vi "Write.vi"(8 "error in (no error)":errorcluster, 11 "UI VISA Terminal in":refnum<class "UI VISA Terminal.lvclass">) -> (0 "error out":errorcluster, 3 "UI VISA Terminal out":refnum<class "UI VISA Terminal.lvclass">)   [LabVIEW 2025, in "UI VISA Terminal.lvlib" / "UI VISA Terminal.lvclass"]
uses:
  UI VISA Terminal.lvclass
  UI VISA Terminal.lvclass/UI VISA Terminal.ctl
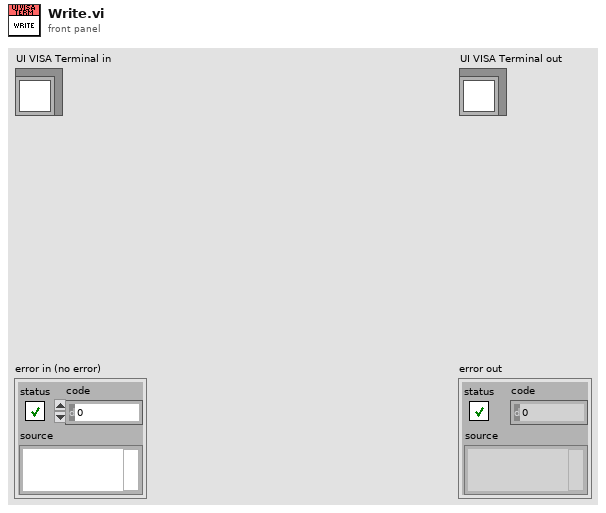
[diagram p1: front panel]
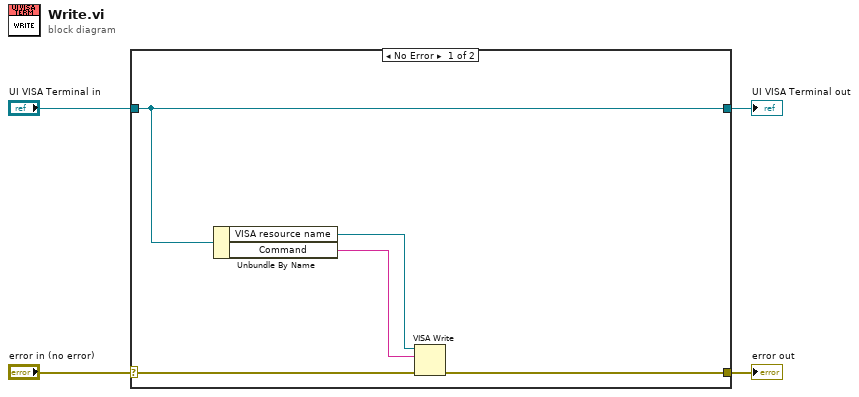
[diagram p0: block diagram]
diagram:
  n1 = case shown="No Error" "error in (no error)" {
    selector: "error in (no error)" -> [w9 w11]
    tunnel: [w8 w11] -> w3
    tunnel: [w7 w10] -> w1
    tunnel: "UI VISA Terminal in" -> [w7 w10]
    frame No Error {
      n2 = Unbundle By Name(w7) -> ("VISA resource name"=w6:refnum<visa-resource-name>, "Command"=w5:string)
      n3 = VISA Write(VISA resource name=w6, write buffer=w5, error in (no error)=w9) -> (error out=w8:errorcluster)  [unwired: 2 out]
    }
    frame Error {
    }
  }
  "error out" <- w3
  "UI VISA Terminal out" <- w1
